vi "Simple Controller.vi"(9 "VISA resource name":refnum<visa-resource-name>="COM10") -> (10 "Starboard Speed":i32(knob) scale=1000.0..2000.0, 11 "Port Speed":i32(knob) scale=1000.0..2000.0)   [LabVIEW 2012]
uses:
  <vilib>/Utility/inputDevices.llb/closeKeyboard.vi
  <vilib>/Utility/inputDevices.llb/keyboardAcquire.vi
panel:
  out "Speed Balance":i32(knob) scale=-1000.0..1000.0
  out "IR Volts":dbl
  in  "ESTOP":bool
  in  "Step Size":i32=5
  in  "PC Status":i32=1
  in  "Pan Camera":i32(slide)=1500 scale=500.0..2500.0
  out "Starboard\nMotor":i32
  out "Port\nMotor":i32
  in  "Rudders":i32(slide)=1500 scale=500.0..2500.0
  out "Right Rubber":i32
  out "Left Rudder":i32
  out "String Received":string
  out "return count":u32
  out "bytes written":u32
  out "Blinky":bool
  in  "String":string="$CS1500P1500R1500L1500P1500H   1\n"
  in  "stop":bool
  # "This routine steers the boat using differential thurst as well as the rudders."
  # "USE THE ARROW KEYS TO CHANGE THE MOTOR SPEEDS, UP AND DOWN MOVE TOGETHER, LEFT AND RIGHT ARE DIFFERENTIAL"
  # "Direction of thrust"
  # "DRAG THE SLIDERS TO MOVE THE RUDDER ANGLES AND PAN THE CAMERA."
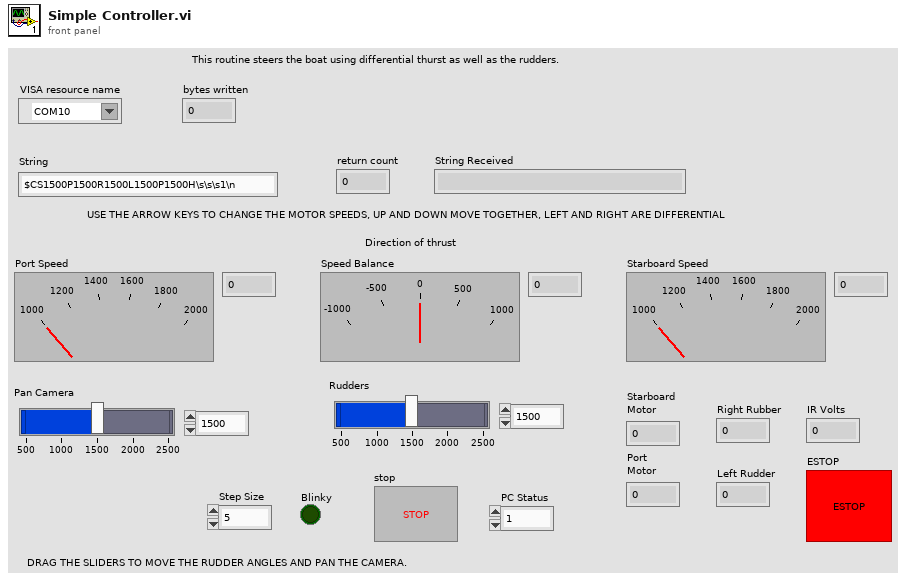
[diagram p1: front panel]
types:
  T1 = enum16{"0", "1", "2", "3", "4", "5", "6", "7", "8", "9", "A", "B", "C", "D", "E", "F", "G", "H", "I", "J", "K", "L", "M", "N", "O", "P", "Q", "R", "S", "T", "U", "V", "W", "X", "Y", "Z", "F1", "F2", "F3", "F4", "F5", "F6", "F7", "F8", "F9", "F10", "F11", "F12", "F13", "F14", "F15", "ADD", "BACK", "BACKSLASH", "CAPITAL", "COMMA", "DECIMAL", "DELETE", "DIVIDE", "DOWN", "END", "EQUALS", "ESCAPE", "GRAVE (`)", "HOME", "INSERT", "LBRACKET", "LCONTROL", "LEFT", "L ALT", "LSHIFT", "LWIN", "MINUS", "MULTIPLY", "NEXT", "NUMLOCK", "NUMPAD_0", "NUMPAD_1", "NUMPAD_2", "NUMPAD_3", "NUMPAD_4", "NUMPAD_5", "NUMPAD_6", "NUMPAD_7", "NUMPAD_8", "NUMPAD_9", "PAUSE", "PERIOD", "PRIOR (PG UP)", "RBRACKET", "RCONTROL", "RETURN", "RIGHT", "R ALT", "RSHIFT", "RWIN", "SCROLL", "SEMICOLON", "SLASH", "SPACE", "SUBTRACT", "TAB", "UP", "ENTER (num pad)", "' (quote)"}[]
  T2 = enum16{"0", "1", "2", "3", "4", "5", "6", "7", "8", "9", "A", "B", "C", "D", "E", "F", "G", "H", "I", "J", "K", "L", "M", "N", "O", "P", "Q", "R", "S", "T", "U", "V", "W", "X", "Y", "Z", "F1", "F2", "F3", "F4", "F5", "F6", "F7", "F8", "F9", "F10", "F11", "F12", "F13", "F14", "F15", "ADD", "BACK", "BACKSLASH", "CAPITAL", "COMMA", "DECIMAL", "DELETE", "DIVIDE", "DOWN", "END", "EQUALS", "ESCAPE", "GRAVE (`)", "HOME", "INSERT", "LBRACKET", "LCONTROL", "LEFT", "L ALT", "LSHIFT", "LWIN", "MINUS", "MULTIPLY", "NEXT", "NUMLOCK", "NUMPAD_0", "NUMPAD_1", "NUMPAD_2", "NUMPAD_3", "NUMPAD_4", "NUMPAD_5", "NUMPAD_6", "NUMPAD_7", "NUMPAD_8", "NUMPAD_9", "PAUSE", "PERIOD", "PRIOR (PG UP)", "RBRACKET", "RCONTROL", "RETURN", "RIGHT", "R ALT", "RSHIFT", "RWIN", "SCROLL", "SEMICOLON", "SLASH", "SPACE", "SUBTRACT", "TAB", "UP", "ENTER (num pad)", "' (quote)"}
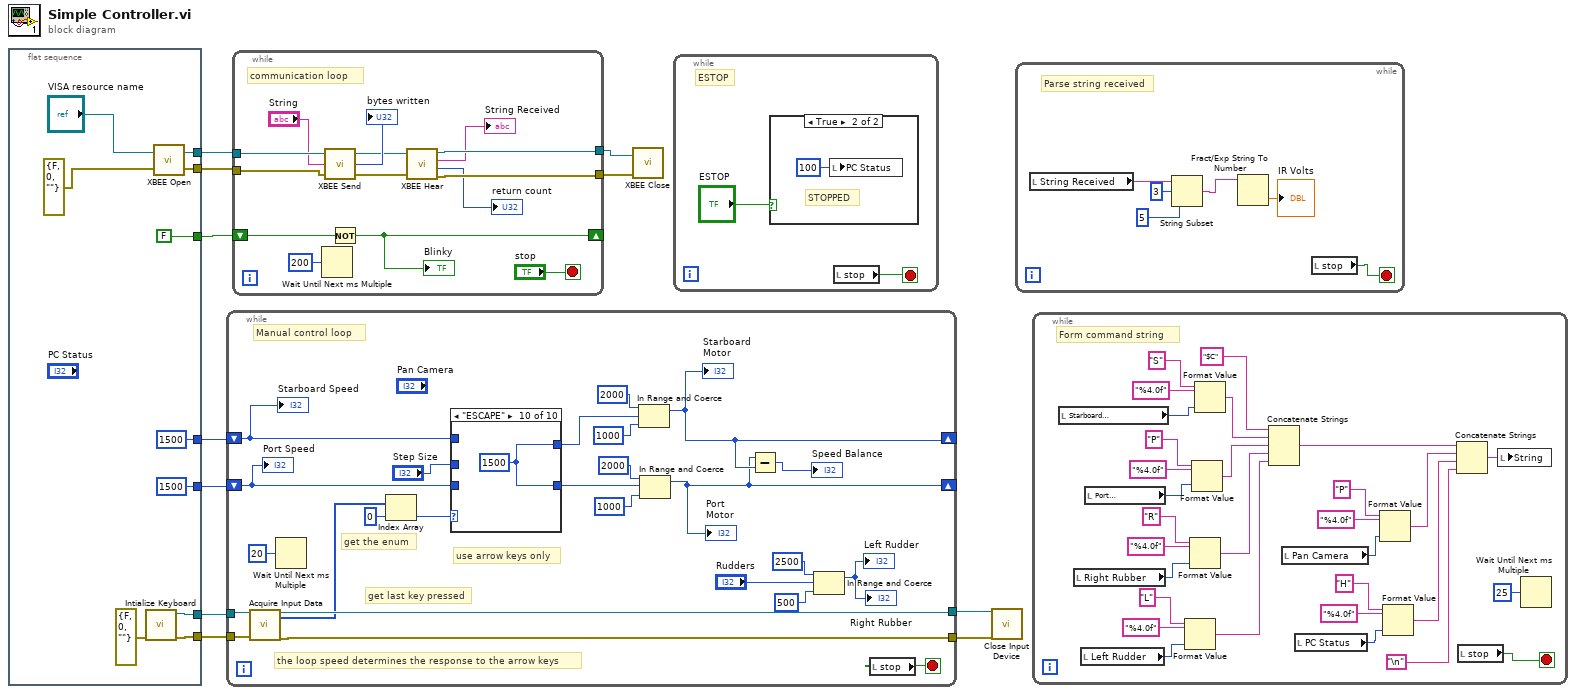
[diagram p0: block diagram]
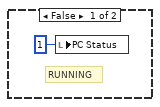
[diagram p2: hidden frame]
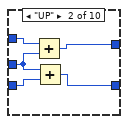
[diagram p4: hidden frame]
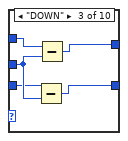
[diagram p5: hidden frame]
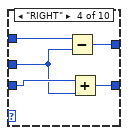
[diagram p6: hidden frame]
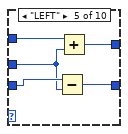
[diagram p7: hidden frame]
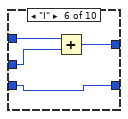
[diagram p8: hidden frame]
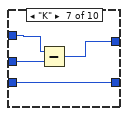
[diagram p9: hidden frame]
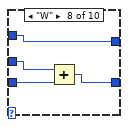
[diagram p10: hidden frame]
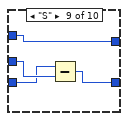
[diagram p11: hidden frame]
diagram:
  n1 = flat-sequence {
    tunnel: [w21] -> w11
    tunnel: [w20] -> w10
    tunnel: [FALSE] -> w7
    tunnel: [w18] -> w6
    tunnel: [w16] -> w5
    tunnel: [1500] -> w2
    tunnel: [1500] -> w1
    frame #0 {
      n2 = call <vilib>:"Intialize Keyboard.vi"("error in (no error)"=errorcluster {"status"=FALSE, "code"=0, "source"=""}) -> ("error out"=w18:errorcluster, "device ID"=w16:refnum<k1>)  [unwired: 9 in]
      n3 = call "XBEE Open.vi"("error in"=errorcluster {"status"=FALSE, "code"=0, "source"=""}, "VISA resource name"="VISA resource name") -> ("error out"=w20:errorcluster, "VISA resource name out"=w21:refnum<visa-resource-name>)
    }
  }
  n4 = while {
    tunnel: w6 -> [w46]
    tunnel: w5 -> [w45]
    tunnel: [w44] -> w4
    tunnel: [w43] -> w3
    shift-right: [w23] -> _
    shift-left: w1 -> [w38]
    shift-right: [w22] -> _
    shift-left: w2 -> [w37]
    stop <- w29 stop-if-true
    # "use arrow keys only"
    # "Manual control loop"
    # "get the enum"
    # "the loop speed determines the response to the arrow keys"
    # "get last key pressed"
    n5 = call-poly <vilib>:"Acquire Input Data.vi"("device ID"=w45, "error in (no error)"=w46) -> ("device ID"=w43:refnum<k1>, "keys pressed"=w42:T1, "error out"=w44:errorcluster)  [unwired: 15 in]
    n6 = Wait Until Next ms Multiple(millisecond multiple=u32 20) -> ()  [unwired: 1 out]
    n7 = Index Array(array=w42, index=0) -> (element=w40:T2)
    n8 = case shown="\"ESCAPE\"" w40 {
      tunnel: w38 -> [w48 w53 w58 w60 w65 w72 w74 w77 w81 _]
      tunnel: [w48 w52 w57 w61 w66 w71 w73 w77 w81 w85] -> w36
      tunnel: w37 -> [w47 w50 w55 w63 w67 w69 w76 w79 w83 _]
      tunnel: [w47 w49 w54 w62 w68 w69 w76 w78 w82 w85] -> w25
      tunnel: "Step Size" -> [_ w51 w56 w59 w64 w70 w75 w80 w84 _]
      frame "0", Default {
      }
      frame "UP" {
        n9 = Add(x=w53, y=w51) -> (x+y=w52:i32)
        n10 = Add(x=w51, y=w50) -> (x+y=w49:i32)
      }
      frame "DOWN" {
        n11 = Subtract(x=w55, y=w56) -> (x-y=w54:i32)
        n12 = Subtract(x=w58, y=w56) -> (x-y=w57:i32)
      }
      frame "RIGHT" {
        n13 = Subtract(x=w60, y=w59) -> (x-y=w61:i32)
        n14 = Add(x=w63, y=w59) -> (x+y=w62:i32)
      }
      frame "LEFT" {
        n15 = Subtract(x=w67, y=w64) -> (x-y=w68:i32)
        n16 = Add(x=w65, y=w64) -> (x+y=w66:i32)
      }
      frame "I" {
        n17 = Add(x=w72, y=w70) -> (x+y=w71:i32)
      }
      frame "K" {
        n18 = Subtract(x=w74, y=w75) -> (x-y=w73:i32)
      }
      frame "W" {
        n19 = Add(x=w80, y=w79) -> (x+y=w78:i32)
      }
      frame "S" {
        n20 = Subtract(x=w83, y=w84) -> (x-y=w82:i32)
      }
      frame "ESCAPE" {
        w85 = 1500
      }
    }
    n21 = In Range and Coerce(upper limit=2000, x=w36, lower limit=1000) -> (coerced(x)=w23:i32)  [unwired: 1 out]
    "Starboard\nMotor" <- w23
    n22 = In Range and Coerce(upper limit=2000, x=w25, lower limit=1000) -> (coerced(x)=w22:i32)  [unwired: 1 out]
    "Port\nMotor" <- w22
    n23 = Subtract(x=w22, y=w23) -> (x-y=→"Speed Balance":i32)
    n24 = In Range and Coerce(upper limit=2500, x="Rudders", lower limit=500) -> (coerced(x)=→"Right Rubber" →"Left Rudder":i32)  [unwired: 1 out]
    n25 = local read "stop"() -> (w29:bool)
    "Starboard Speed" <- w38
    "Port Speed" <- w37
  }
  n26 = while {
    tunnel: w11 -> [w98]
    tunnel: w10 -> [w97]
    tunnel: [w92] -> w9
    tunnel: [w91] -> w8
    shift-right: [w95] -> _
    shift-left: w7 -> [w96]
    stop <- "stop" stop-if-true
    # "communication loop"
    n27 = Wait Until Next ms Multiple(millisecond multiple=u32 200) -> ()  [unwired: 1 out]
    n28 = call "XBEE Send.vi"("error in (no error)"=w97, "String"="String", "VISA resource name"=w98) -> ("error out"=w88:errorcluster, "return count"=→"bytes written":u32, "VISA resource name out"=w89:refnum<visa-resource-name>)
    n29 = Not(x=w96) -> (.not. x?=w95:bool)
    "Blinky" <- w95
    n30 = call "XBEE Hear.vi"("VISA resource name"=w89, "error in (no error)"=w88) -> ("VISA resource name out"=w92:refnum<visa-resource-name>, "String Received"=→"String Received":string, "return count"=→"return count":u32, "error out"=w91:errorcluster)
  }
  n31 = call "XBEE Close.vi"("error in (no error)"=w8, "VISA resource name"=w9) -> ()
  n32 = while {
    stop <- w101 stop-if-true
    # "ESTOP"
    n33 = case shown="True" "ESTOP" {
      frame False {
        # "RUNNING"
        n34 = local write "PC Status"(1 ("PC Status")) -> ()
      }
      frame True {
        # "STOPPED"
        n35 = local write "PC Status"(100) -> ()
      }
    }
    n36 = local read "stop"() -> (w101:bool)
  }
  n37 = call-poly <vilib>:"Close Input Device.vi"("error in (no error)"=w4, "device ID"=w3) -> ()  [unwired: 8 in, 1 out]
  n38 = while {
    stop <- w106 stop-if-true
    # "Parse string received"
    n39 = local read "String Received"() -> (w109:string)
    n40 = String Subset(string=w109, offset (0)=3, length (rest)=5 ("length (rest)")) -> (substring=w105:string)
    n41 = Fract/Exp String To Number(string=w105) -> (number=→"IR Volts":dbl)  [unwired: 3 in, 1 out]
    n42 = local read "stop"() -> (w106:bool)
  }
  n43 = while {
    stop <- w139 stop-if-true
    # "Form command string"
    n44 = local read "Starboard\nMotor"() -> (w136:i32)
    n45 = local read "Right Rubber"() -> (w127:i32)
    n46 = local read "Left Rudder"() -> (w124:i32)
    n47 = local read "Port\nMotor"() -> (w133:i32)
    n48 = Format Value(string ("")="L", format string="%4.0f", value (0)=w124) -> (output string=w122:string)
    n49 = Format Value(string ("")="R", format string="%4.0f", value (0)=w127) -> (output string=w123:string)
    n50 = Format Value(string ("")="P", format string="%4.0f", value (0)=w133) -> (output string=w130:string)
    n51 = Format Value(string ("")="S", format string="%4.0f", value (0)=w136) -> (output string=w131:string)
    n52 = Concatenate Strings("$C", w131, w130, w123, w122) -> (w114:string)
    n53 = local read "Pan Camera"() -> (w118:i32)
    n54 = local read "PC Status"() -> (w115:i32)
    n55 = Format Value(string ("")="P", format string="%4.0f", value (0)=w118) -> (output string=w113:string)
    n56 = Format Value(string ("")="H", format string="%4.0f", value (0)=w115) -> (output string=w112:string)
    n57 = Concatenate Strings(w114, w113, w112, "\n") -> (w119:string)
    n58 = local read "stop"() -> (w139:bool)
    n59 = local write "String"(w119) -> ()
    n60 = Wait Until Next ms Multiple(millisecond multiple=u32 25) -> ()  [unwired: 1 out]
  }
